vi "test Compile RaF Channel Data With Disabled Channel.vi"(8 "error in (no error)":errorcluster, 11 "TestCase in":refnum<class "Routing and Faulting Compile Unit Tests.lvclass">) -> (0 "error out":errorcluster, 3 "TestCase out":refnum<class "Routing and Faulting Compile Unit Tests.lvclass">)   [LabVIEW 2020, in "Routing and Faulting Compile Unit Tests.lvclass"]
uses:
  Routing and Faulting Compile Unit Tests.lvclass
  Shared/Channel States.ctl
  Shared/Routing State.ctl
  Shared/Connection.ctl
  Shared/Compiled.Settings.ctl
  Shared/Communication Configuration.ctl
  Shared/Routing and Faulting Configuration.ctl
  Shared/Routing Channel Configuration.ctl
  Shared/Value-Connections Map.ctl
  Shared/Alias Mapping.ctl
  Shared/Alias Endpoint.ctl
  Shared/Compiled Connection.ctl
  Shared/FIFO Indices.ctl
  Routing and Faulting Compile Unit Tests.lvclass/Routing and Faulting Compile Unit Tests.ctl
  System Explorer/Get Channel Data in By Channel ID (offline).vi
  Scripting/Routing and Faulting Scripting.lvlib
  Shared/Routing and Faulting Shared.lvlib
  System Explorer/Routing and Faulting System Explorer.lvlib
panel:
  in  "Save?":bool
  out "Output Filename":string
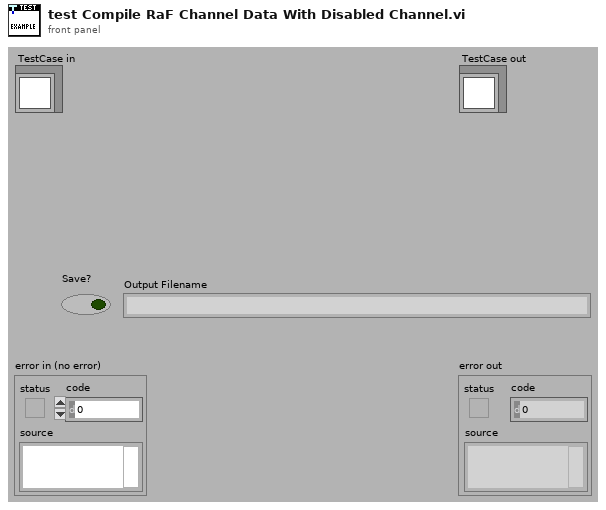
[diagram p1: front panel]
types:
  T1 = typedef "Routing and Faulting Shared.lvlib/Alias Endpoint.ctl" = cluster{"Module Path":string, "Endpoint":string}
  T2 = cluster{"Value-Connections Map.Connection List Array":cluster{"Compiled Connections Indices":i32[]}[]}[]
  T3 = typedef "Routing and Faulting Shared.lvlib/Compiled Connection.ctl" = cluster{"Consumer Queue Index":i32, "Normalized Connection String":string}
  T4 = typedef "Routing and Faulting Shared.lvlib/Communication Configuration.ctl" = cluster{"Consumer Queue Names":string[]}
  T5 = typedef "Routing and Faulting Shared.lvlib/Compiled.Settings.ctl" = cluster{"Custom Device Name":string, "Communication Configuration":T4, "Routing and Faulting Configuration":T6, "Status Channels FIFO Indices":T10}
  T6 = typedef "Routing and Faulting Shared.lvlib/Routing and Faulting Configuration.ctl" = cluster{"Routing Channel Configurations":T7[], "Alias Mappings":T9[], "Compiled Connection Buffer":T3[], "Compiled Initial Connection Indices":i32[]}
  T7 = typedef "Routing and Faulting Shared.lvlib/Routing Channel Configuration.ctl" = cluster{"Channel Name":string, "Initial Value":dbl, "FIFO Index":i32, "Value-Connections Map":T8}
  T8 = typedef "Routing and Faulting Shared.lvlib/Value-Connections Map.ctl" = cluster{"State Value Array":i32[], "Connection List Array":cluster{"Compiled Connections Indices":i32[]}[]}
  T9 = typedef "Routing and Faulting Shared.lvlib/Alias Mapping.ctl" = cluster{"Alias":string, "Endpoint":T1}
  T10 = typedef "Routing and Faulting Shared.lvlib/FIFO Indices.ctl" = cluster{"Status Channel":i32, "Heartbeat Channel":i32}
  T11 = typedef "Routing and Faulting Shared.lvlib/Channel States.ctl" = T12[]
  T12 = typedef "Routing and Faulting Shared.lvlib/Routing State.ctl" = cluster{"Name":string, "Description":string, "Value":i32, "Connection List":T13[]}
  T13 = typedef "Routing and Faulting Shared.lvlib/Connection.ctl" = cluster{"Module":string, "Source":string, "Destination":string}
  T14 = typedef "Custom Device API.lvlib/Custom Device Item Ref.ctl" = u64
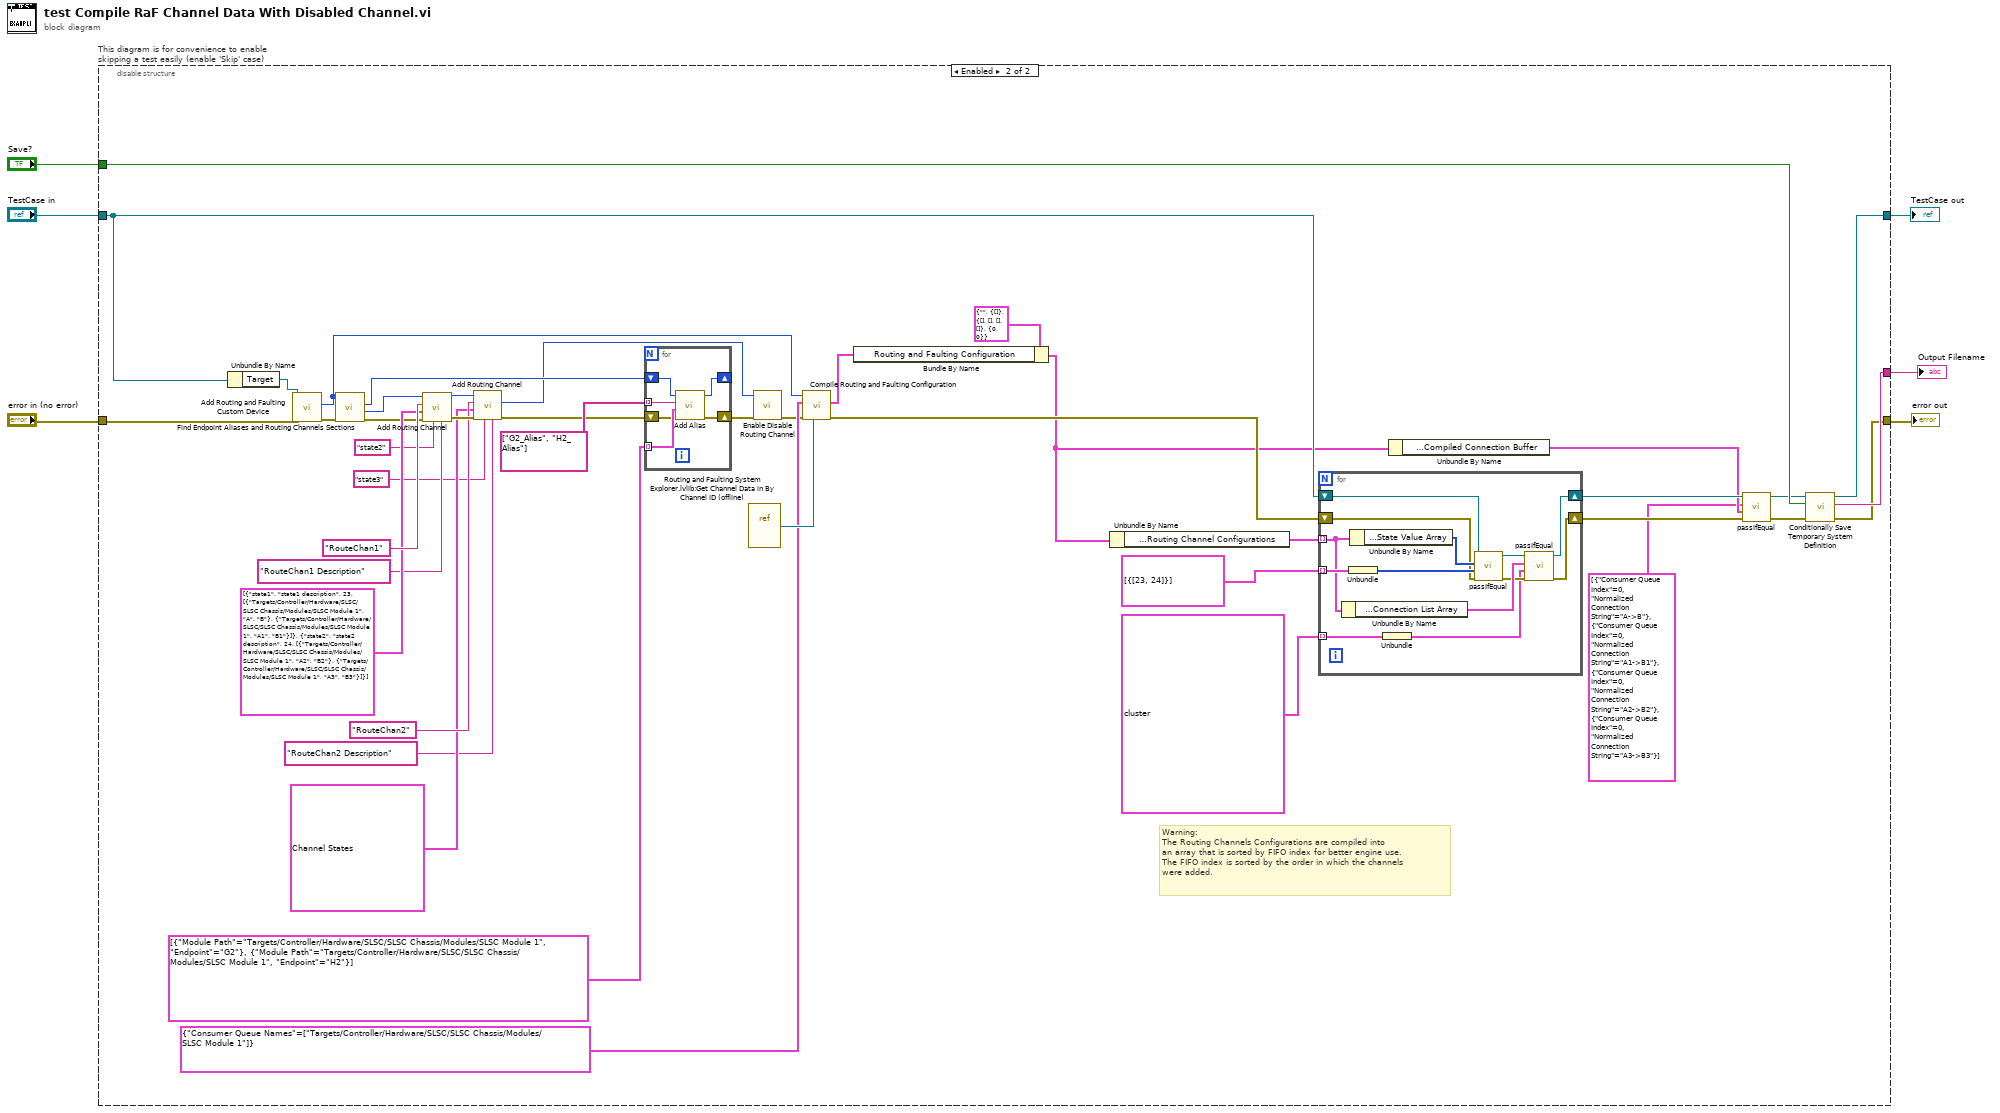
[diagram p0: block diagram]
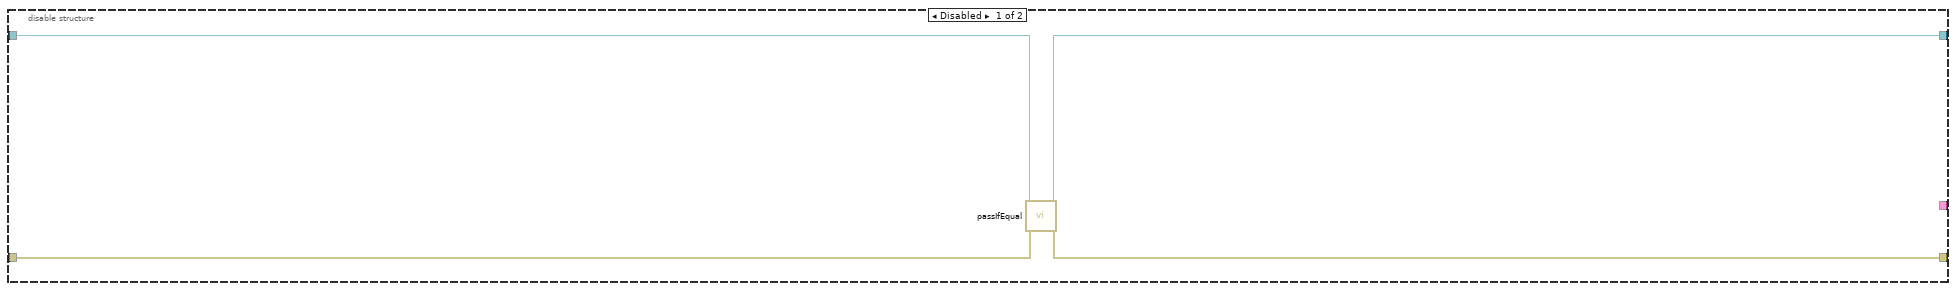
[diagram p2: hidden frame]
diagram:
  n1 = disable-structure "This diagram is for convenience to enable skipping a test easily (enable 'Skip' case)" shown="Enabled" {
    disable-tunnel: "TestCase in" -> [w10 w43]
    disable-tunnel: [w9 w48] -> w3
    disable-tunnel: [w8 w40] -> w5
    disable-tunnel: "error in (no error)" -> [w7 w50]
    disable-tunnel: "Save?" -> [_ w49]
    disable-tunnel: [_ w47] -> w1
    frame Disabled {
      n2 = call-dynamic "passIfEqual.vi"("error in (no error)"=w7, "TestCase in"=w10) -> ("error out"=w8:errorcluster, "TestCase out"=w9:refnum<class "Routing and Faulting Compile Unit Tests.lvclass">)  [unwired: 8 in]
    }
    frame Enabled {
      # "Warning: \nThe Routing Channels Configurations are compiled into\nan array that is sorted by FIFO index for better engine use.\nThe FIFO index is sorted by the order in which the channels\nwere added."
      n3 = Unbundle By Name(w43) -> ("Target"=w51:refnum<k24>)
      n4 = call "Add Routing and Faulting Custom Device.vi"("error in"=w50, "target in"=w51) -> ("error out"=w53:errorcluster, "routing and faulting custom device"=w26:T14)  [unwired: 7 in, 1 out]
      n5 = call "Find Endpoint Aliases and Routing Channels Sections.vi"("error in"=w53, "routing and faulting custom device in"=w26) -> ("error out"=w36:errorcluster, "routing channels"=w35:T14, "endpoint aliases"=w34:T14)  [unwired: 6 in, 1 out]
      n6 = call "Add Routing Channel.vi"("description"="RouteChan1 Description" ("Description"), "initial state"="state2" ("Initial State"), "error in"=w36, "state configurations"=T11 [{"Name"="state1", "Description"="state1 description", "Value"=23, "Connection List"=[{"Module"="Targets/Controller/Hardware/SLSC/SLSC Chassis/Modules/SLSC Module 1", "Source"="A", "Destination"="B"}, {"Module"="Targets/Controller/Hardware/SLSC/SLSC Chassis/Modules/SLSC Module 1", "Source"="A1", "Destination"="B1"}]}, {"Name"="state2", "Description"="state2 description", "Value"=24, "Connection List"=[{"Module"="Targets/Controller/Hardware/SLSC/SLSC Chassis/Modules/SLSC Module 1", "Source"="A2", "Destination"="B2"}, {"Module"="Targets/Controller/Hardware/SLSC/SLSC Chassis/Modules/SLSC Module 1", "Source"="A3", "Destination"="B3"}]}] ("States and Connections"), "channel name"="RouteChan1" ("Channel Name"), "routing channels in"=w35) -> ("error out"=w46:errorcluster, "routing channels out"=w45:T14)  [unwired: 3 in, 1 out]
      n7 = call "Add Routing Channel.vi"("description"="RouteChan2 Description" ("Description"), "initial state"="state3" ("Initial State"), "error in"=w46, "state configurations"=T11 [{"Name"="state3", "Description"="state3 description", "Value"=33, "Connection List"=[{"Module"="Targets/Controller/Hardware/SLSC/SLSC Chassis/Modules/SLSC Module 1", "Source"="G", "Destination"="H"}, {"Module"="Targets/Controller/Hardware/SLSC/SLSC Chassis/Modules/SLSC Module 1", "Source"="G1", "Destination"="G2"}, {"Module"="Targets/Controller/Hardware/SLSC/SLSC Chassis/Modules/SLSC Module 1", "Source"="H2", "Destination"="G2"}]}, {"Name"="state4", "Description"="state4 description", "Value"=34, "Connection List"=[{"Module"="Targets/Controller/Hardware/SLSC/SLSC Chassis/Modules/SLSC Module 1", "Source"="G2", "Destination"="H2"}, {"Module"="Targets/Controller/Hardware/SLSC/SLSC Chassis/Modules/SLSC Module 1", "Source"="G3", "Destination"="H3"}, {"Module"="Targets/Controller/Hardware/SLSC/SLSC Chassis/Modules/SLSC Module 1", "Source"="G4", "Destination"="H4"}]}] ("States and Connections"), "channel name"="RouteChan2" ("Channel Name"), "routing channels in"=w45) -> ("error out"=w38:errorcluster, "routing channel"=w12:T14)  [unwired: 3 in, 1 out]
      n8 = for {
        shift-right: [w56] -> _
        shift-left: w34 -> [w57]
        tunnel: string[] ["G2_Alias", "H2_Alias"] -> [w59] mode=indexing
        tunnel: T1[] [{"Module Path"="Targets/Controller/Hardware/SLSC/SLSC Chassis/Modules/SLSC Module 1", "Endpoint"="G2"}, {"Module Path"="Targets/Controller/Hardware/SLSC/SLSC Chassis/Modules/SLSC Module 1", "Endpoint"="H2"}] -> [w58] mode=indexing
        shift-right: [w55] -> w14
        shift-left: w38 -> [w54]
        n9 = call "Add Alias.vi"("error in"=w54, "endpoint"=w58, "alias"=w59, "endpoint aliases in"=w57) -> ("error out"=w55:errorcluster, "endpoint aliases out"=w56:T14)  [unwired: 6 in]
      }
      n10 = vi-ref "Routing and Faulting System Explorer.lvlib:Get Channel Data in By Channel ID (offline).vi"() -> (w25:refnum<vi>)
      n11 = call "Enable Disable Routing Channel.vi"("error in (no error)"=w14, "Node Ptr"=w12) -> ("error out"=w13:errorcluster)  [unwired: 8 in, 1 out]
      n12 = call "Compile Routing and Faulting Configuration.vi"("Get Channel Data Refnum"=w25, "error in (no error)"=w13, "Communication Configuration"=T4 {"Consumer Queue Names"=["Targets/Controller/Hardware/SLSC/SLSC Chassis/Modules/SLSC Module 1"]}, "Device Ref in"=w26) -> ("error out"=w28:errorcluster, "RaF Configuration"=w27:T6)  [unwired: 5 in, 1 out]
      n13 = Bundle By Name(cluster=T5 {"Custom Device Name"="", "Communication Configuration"={"Consumer Queue Names"=[]}, "Routing and Faulting Configuration"={"Routing Channel Configurations"=[], "Alias Mappings"=[], "Compiled Connection Buffer"=[], "Compiled Initial Connection Indices"=[]}, "Status Channels FIFO Indices"={"Status Channel"=0, "Heartbeat Channel"=0}} ("Compiled.Settings.ctl"), "Routing and Faulting Configuration"=w27) -> (w21:T5)
      n14 = Unbundle By Name(w21) -> ("Routing and Faulting Configuration.Routing Channel Configurations"=w22:T7[])
      n15 = for {
        tunnel: w22 -> [w68] mode=indexing
        tunnel: cluster{i32[]}[] [{[23, 24]}] ("expected State Values") -> [w72] mode=indexing
        shift-right: [w65] -> w19
        shift-left: w43 -> [w64]
        shift-right: [w62] -> w20
        shift-left: w28 -> [w63]
        tunnel: T2 [{"Value-Connections Map.Connection List Array"=[{"Compiled Connections Indices"=[0, 1]}, {"Compiled Connections Indices"=[2, 3]}]}] -> [w61] mode=indexing
        n16 = Unbundle By Name(w68) -> ("Value-Connections Map.Connection List Array"=w69:cluster{"Compiled Connections Indices":i32[]}[])
        n17 = Unbundle(w72) -> (w71:i32[])
        n18 = Unbundle By Name(w68) -> ("Value-Connections Map.State Value Array"=w70:i32[])
        n19 = Unbundle(w61) -> ("Value-Connections Map.Connection List Array"=w60:cluster{"Compiled Connections Indices":i32[]}[])
        n20 = call-dynamic "passIfEqual.vi"("error in (no error)"=w63, "y"=w71, "x"=w70, "TestCase in"=w64) -> ("error out"=w67:errorcluster, "TestCase out"=w66:refnum<class "Routing and Faulting Compile Unit Tests.lvclass">)  [unwired: 6 in]
        n21 = call-dynamic "passIfEqual.vi"("error in (no error)"=w67, "y"=w60, "x"=w69, "TestCase in"=w66) -> ("error out"=w62:errorcluster, "TestCase out"=w65:refnum<class "Routing and Faulting Compile Unit Tests.lvclass">)  [unwired: 6 in]
      }
      n22 = Unbundle By Name(w21) -> ("Routing and Faulting Configuration.Compiled Connection Buffer"=w16:T3[])
      n23 = call-dynamic "passIfEqual.vi"("error in (no error)"=w20, "y"=w16, "x"=T3[] [{"Consumer Queue Index"=0, "Normalized Connection String"="A->B"}, {"Consumer Queue Index"=0, "Normalized Connection String"="A1->B1"}, {"Consumer Queue Index"=0, "Normalized Connection String"="A2->B2"}, {"Consumer Queue Index"=0, "Normalized Connection String"="A3->B3"}] ("Routing and Faulting Configuration.Compiled Connection Buffer"), "TestCase in"=w19) -> ("error out"=w17:errorcluster, "TestCase out"=w18:refnum<class "Routing and Faulting Compile Unit Tests.lvclass">)  [unwired: 6 in]
      n24 = call "Conditionally Save Temporary System Definition.vi"("error in (no error)"=w17, "Save?"=w49, "TestCase in"=w18) -> ("error out"=w40:errorcluster, "filename"=w47:string, "TestCase out"=w48:refnum<class "Routing and Faulting Compile Unit Tests.lvclass">)  [unwired: 6 in]
    }
  }
  "error out" <- w5
  "TestCase out" <- w3
  "Output Filename" <- w1
